vi "1poputkapechat (SubVI).vi"(11 "Protocol in":string[][](table)=[["11.02.26 11:54:00", "3.0012e-3", "3.0012e-3", "125,65", "125,65", "1 В", "1 В"], ["", "", "", "", "", "", ""]]) -> ()   [LabVIEW 2017]
uses:
  <vilib>/Utility/file.llb/Write Delimited Spreadsheet (string).vi
  <vilib>/Utility/NIReport.llb/Append Report Text (str wrap).vi
  <vilib>/Utility/NIReport.llb/NI_report.lvclass
panel:
  in  "Boolean":bool
  in  "MS Office parameters":T1
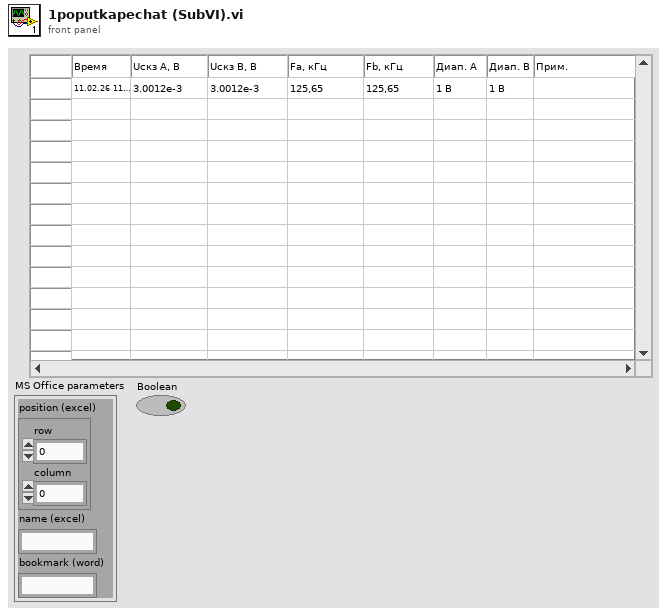
[diagram p1: front panel]
types:
  T1 = cluster{"position (excel)":cluster{"row":i32, "column":i32}, "name (excel)":string, "bookmark (word)":string}
  T2 = enum16{"Standard Report", "HTML", "Word", "Excel"}
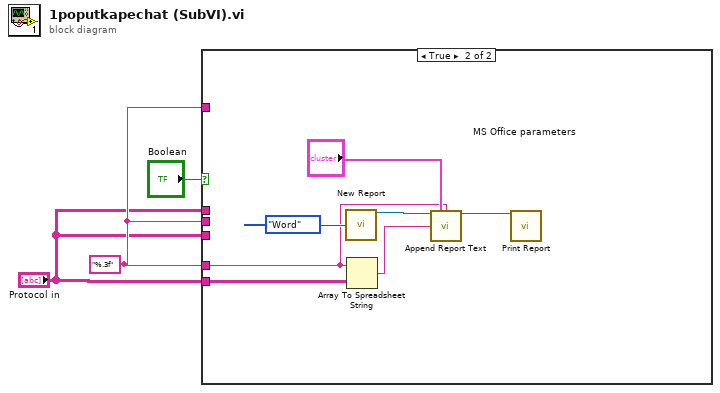
[diagram p0: block diagram]
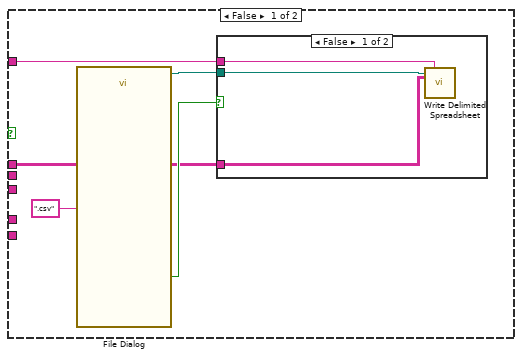
[diagram p2: hidden frame]
diagram:
  w2 = "%.3f" ("delimiter (Tab)")
  n1 = case shown="True" "Boolean" {
    tunnel: "Protocol in" -> [_ w13]
    tunnel: w2 -> [_ w12]
    tunnel: w2 -> [_ _]
    tunnel: "Protocol in" -> [_ _]
    tunnel: w2 -> [w7 _]
    tunnel: "Protocol in" -> [w6 _]
    frame False {
      n2 = call "File Dialog"("pattern (all files)"=".csv") -> ("selected path"=w5:path, "cancelled"=w8:bool)  [unwired: 11 in, 2 out]
      n3 = case shown="False" w8 {
        tunnel: w7 -> [w11 _]
        tunnel: w6 -> [w10 _]
        tunnel: w5 -> [w9 _]
        frame False {
          n4 = call-poly <vilib>:"Write Delimited Spreadsheet.vi"("file path (dialog if empty)"=w9, "format (%s)"=w11, "2D data"=w10) -> ()  [unwired: 11 in, 2 out]
        }
        frame True {
        }
      }
    }
    frame True {
      n5 = call <vilib>:"New Report.vi"("report type"=T2."Word") -> ("report out"=w16:refnum<class "NI_report.lvclass">)  [unwired: 13 in, 1 out]
      n6 = Array To Spreadsheet String(array=w13, 3:w12) -> (spreadsheet string=w17:string)  [unwired: 1 in]
      n7 = call-poly <vilib>:"Append Report Text.vi"("report in"=w16, "MS Office parameters"="MS Office parameters", "format string (%.3f)"=w12, "text"=w17) -> ("report out"=w15:refnum<class "NI_report.lvclass">)  [unwired: 8 in, 3 out]
      n8 = call-dynamic "Print Report.vi"("report in"=w15) -> ()  [unwired: 13 in, 2 out]
    }
  }
